vi "run.vi"() -> ()   [LabVIEW 2017]
panel:
  out "Array 2":i32[](array[numeric])
  out "Array":i32[](array[numeric])
  out "sum":i64
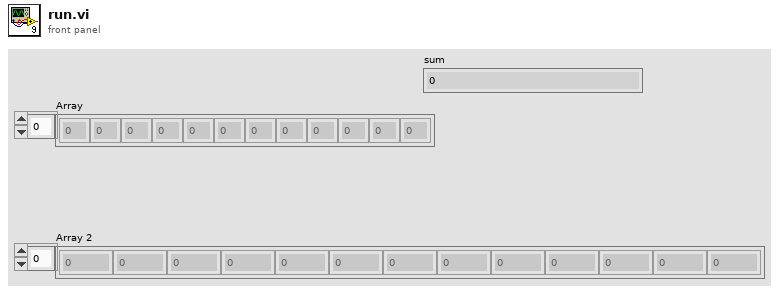
[diagram p1: front panel]
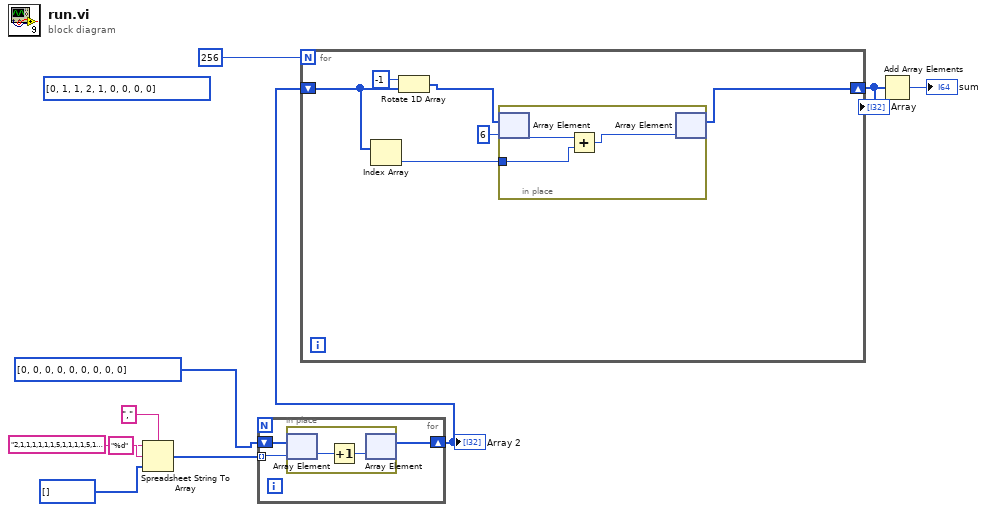
[diagram p0: block diagram]
diagram:
  (unwired) i64[] [0, 1, 1, 2, 1, 0, 0, 0, 0]
  n1 = Spreadsheet String To Array(delimiter (Tab)=",", format string="%d", spreadsheet string="2,1,1,1,1,1,1,5,1,1,1,1,5,1,1,3,5,1,1,3,1,1,3,1,4,4,4,5,1,1,1,3,1,3,1,1,2,2,1,1,1,5,1,1,1,5,2,5,1,1,2,1,3,3,5,1,1,4,1,1,3,1,1,1,1,1,1,1,1,1,1,1,1,4,1,5,1,2,1,1,1,1,5,1,1,1,1,1,5,1,1,1,4,5,1,1,3,4,1,1,1,3,5,1,1,1,2,1,1,4,1,4,1,2,1,1,2,1,5,1,1,1,5,1,2,2,1,1,1,5,1,2,3,1,1,1,5,3,2,1,1,3,1,1,3,1,3,1,1,1,5,1,1,1,1,1,1,1,3,1,1,1,1,3,1,1,4,1,1,3,2,1,2,1,1,2,2,1,2,1,1,1,4,1,2,4,1,1,4,4,1,1,1,1,1,4,1,1,1,2,1,1,2,1,5,1,1,1,1,1,5,1,3,1,1,2,3,4,4,1,1,1,3,2,4,4,1,1,3,5,1,1,1,1,4,1,1,1,1,1,5,3,1,5,1,1,1,1,1,1,1,1,1,1,1,1,1,1,1,1,1,1,1,1,5,1,1,1,1,1,1,1,1,5,1,4,4,1,1,1,1,1,1,1,1,3,1,3,1,4,1,1,2,2,2,1,1,2,1,1", array type (2D Dbl)=i32[] []) -> (array=w3:i32[])
  n2 = for {
    tunnel: w3 -> [w12] mode=indexing
    shift-right: [w11] -> w1
    shift-left: i64[] [0, 0, 0, 0, 0, 0, 0, 0, 0] -> [w13]
    n3 = in-place {
      n4 = in-place-array #1(w13, w12) -> (w15:i64)
      n5 = Increment(x=w15) -> (x+1=w14:i64)
      n6 = in-place-array #1(w14) -> (w11:i64[])  [unwired: 1 out]
    }
  }
  "Array 2" <- w1
  n7 = for {
    N: 256 -> [_]
    shift-right: [w18] -> w9
    shift-left: w1 -> [w17]
    n8 = Index Array(array=w17) -> (element=w16:i64)  [unwired: 1 in]
    n9 = Rotate 1D Array(1:w17, 2:-1 ("n")) -> (0:w19:i64[])
    n10 = in-place {
      in-place-border: w16 -> [w23]
      n11 = in-place-array #2(w19, 6) -> (w24:i64)
      n12 = Add(x=w24, y=w23) -> (x+y=w22:i64)
      n13 = in-place-array #2(w22) -> (w18:i64[])  [unwired: 1 out]
    }
  }
  "Array" <- w9
  n14 = Add Array Elements(numeric array=w9) -> (sum=→"sum":i64)
